vi "GetXMLTagRobust.vi"(0 "Tag only? (T)":bool=TRUE, 1 "Tag":string, 2 "String":string) -> (3 "value":string, 4 "Correct Tag Exists?":bool, 5 "tag found":string, 6 "String w/o Tag":string)   [LabVIEW 2015]
uses:
  vi.lib/regexp/Match Regular Expression.xnode
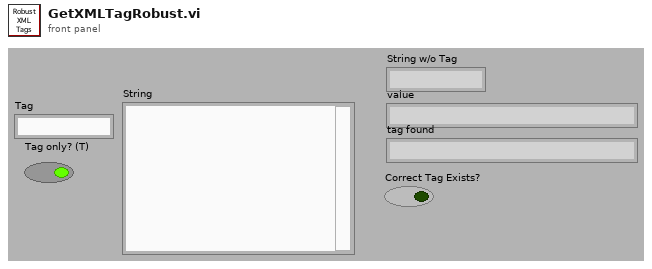
[diagram p1: front panel]
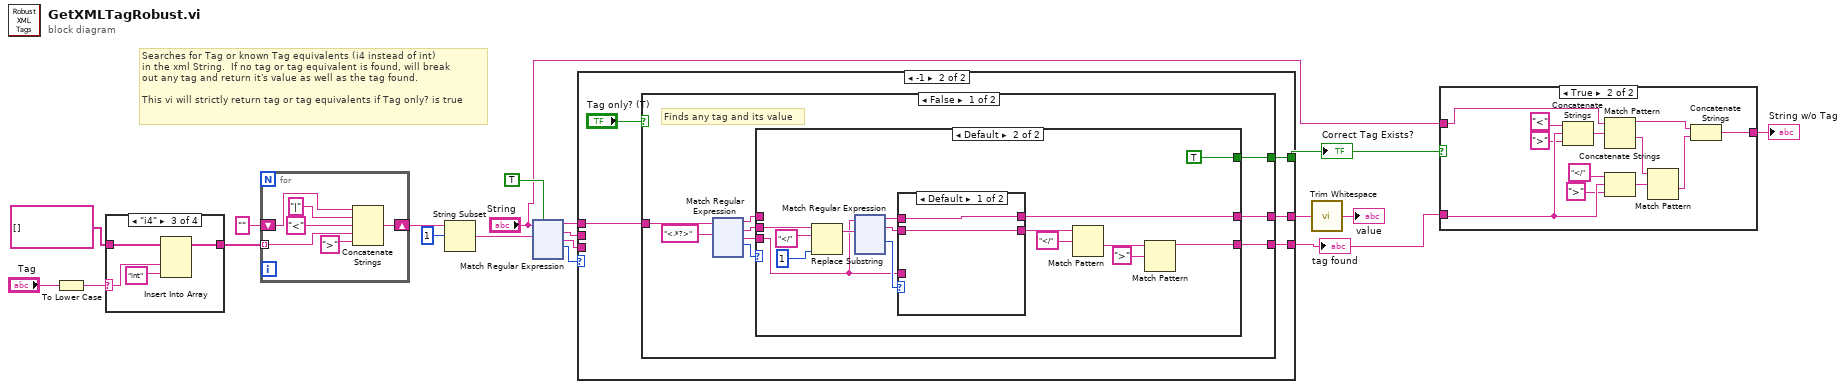
[diagram p0: block diagram]
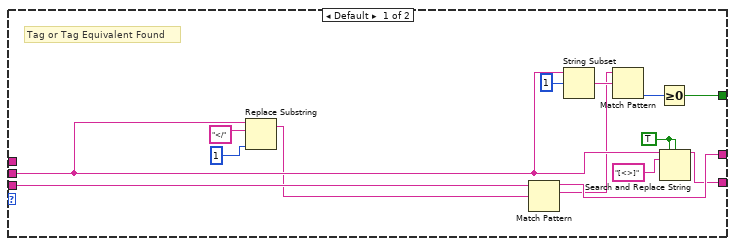
[diagram p3: hidden frame]
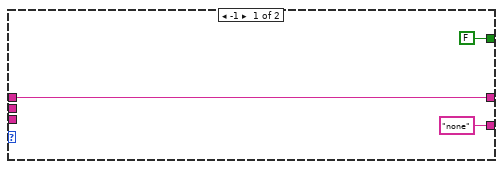
[diagram p4: hidden frame]
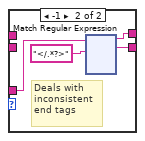
[diagram p5: hidden frame]
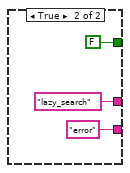
[diagram p6: hidden frame]
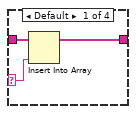
[diagram p7: hidden frame]
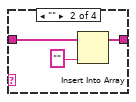
[diagram p8: hidden frame]
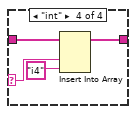
[diagram p9: hidden frame]
diagram:
  # "Searches for Tag or known Tag equivalents (i4 instead of int)\nin the xml String.  If no tag or tag equivalent is found, will break\nout any tag and return it's value as well as the tag found.\n\nThis vi will strictly return tag or tag equivalents if Tag only? is true"
  n1 = To Lower Case(string="Tag") -> (all lower case string=w7:string)
  n2 = case shown="\"i4\"" w7 {
    selector: w7 -> [w20 _ w26 w30]
    tunnel: string[] [] -> [w22 w25 w29 w33]
    tunnel: [w21 w24 w28 w32] -> w18
    frame Default {
      n3 = Insert Into Array(array=w22, new element=w20) -> (w21:string[])  [unwired: 1 in]
    }
    frame "" {
      n4 = Insert Into Array(array=w25, new element="" ("new element/subarray")) -> (w24:string[])  [unwired: 1 in]
    }
    frame "i4" {
      n5 = Insert Into Array(array=w29, new element #1=w26, new element #2="int" ("new element/subarray")) -> (w28:string[])  [unwired: 1 in]
    }
    frame "int" {
      n6 = Insert Into Array(array=w33, new element #1=w30, new element #2="i4" ("new element/subarray")) -> (w32:string[])  [unwired: 1 in]
    }
  }
  n7 = for {
    tunnel: w18 -> [w36] mode=indexing
    shift-right: [w37] -> w16
    shift-left: "" -> [w39]
    n8 = Concatenate Strings(w39, "|" ("string"), "<" ("string"), w36, ">" ("string")) -> (w37:string)
  }
  n9 = String Subset(string=w16, offset (0)=1) -> (substring=w14:string)  [unwired: 1 in]
  n10 = xnode "Match Regular Expression"("input string"="String", "regular expression"=w14, "ignore case? (F)"=TRUE) -> ("before match"=w13:string, "whole match"=w10:string, "after match"=w9:string, "offset past match"=w12:i32)  [unwired: 3 in, 1 out]
  n11 = case shown="-1" w12 {
    tunnel: w13 -> [_ w58]
    tunnel: w10 -> [w42 _]
    tunnel: w9 -> [w50 _]
    tunnel: [w53 w57] -> w6
    tunnel: [w49 w56] -> w1
    tunnel: [w51 w55] -> w4
    frame Default {
      w47 = TRUE ("replace all? (F)")
      # "Tag or Tag Equivalent Found"
      n12 = Replace Substring(2:1 ("length (len. of substring)"), 4:"</" ("substring (\"\")"), 5:w42) -> (1:w41:string)  [unwired: 1 in, 1 out]
      n13 = Match Pattern(string=w50, regular expression=w41) -> (before substring=w53:string, match substring=w40:string)  [unwired: 1 in, 2 out]
      n14 = String Subset(string=w42, offset (0)=1) -> (substring=w45:string)  [unwired: 1 in]
      n15 = Match Pattern(string=w40, regular expression=w45) -> (offset past match=w52:i32)  [unwired: 1 in, 3 out]
      n16 = Greater Or Equal To 0?(x=w52) -> (x >= 0?=w51:bool)
      n17 = Search and Replace String(replace all?=w47, case sensitive?=w47, input string=w42, search string="[<>]") -> (result string=w49:string)  [unwired: 4 in, 3 out]
    }
    frame -1 {
      n18 = case shown="False" "Tag only? (T)" {
        tunnel: w58 -> [w66 _]
        tunnel: [w63 "lazy_search" ("before match")] -> w57
        tunnel: [w62 "error" ("whole match")] -> w56
        tunnel: [w60 FALSE] -> w55
        frame False {
          # "Finds any tag and its value"
          n19 = xnode "Match Regular Expression"("input string"=w66, "regular expression"="<.*?>") -> ("before match"=w61:string, "whole match"=w59:string, "after match"=w65:string, "offset past match"=w64:i32)  [unwired: 4 in, 1 out]
          n20 = case shown="Default" w64 {
            tunnel: w65 -> [_ w75]
            tunnel: [w69 w74] -> w63
            tunnel: ["none" ("whole match") w82] -> w62
            tunnel: w61 -> [w69 _]
            tunnel: [FALSE TRUE] -> w60
            tunnel: w59 -> [_ w80]
            frame -1 {
            }
            frame Default {
              n21 = Replace Substring(2:1 ("length (len. of substring)"), 4:"</" ("substring (\"\")"), 5:w80) -> (1:w77:string)  [unwired: 1 in, 1 out]
              n22 = xnode "Match Regular Expression"("input string"=w75, "regular expression"=w77) -> ("before match"=w72:string, "whole match"=w71:string, "offset past match"=w76:i32)  [unwired: 4 in, 2 out]
              n23 = case shown="Default" w76 {
                tunnel: w75 -> [_ w91]
                tunnel: [w87 w89] -> w74
                tunnel: [w86 w88] -> w73
                tunnel: w72 -> [w87 _]
                tunnel: w71 -> [w86 _]
                frame Default {
                }
                frame -1 {
                  # "Deals with\ninconsistent \nend tags"
                  n24 = xnode "Match Regular Expression"("input string"=w91, "regular expression"="</.*?>") -> ("before match"=w89:string, "whole match"=w88:string)  [unwired: 4 in, 3 out]
                }
              }
              n25 = Match Pattern(string=w73, regular expression="</") -> (after substring=w84:string)  [unwired: 1 in, 3 out]
              n26 = Match Pattern(string=w84, regular expression=">") -> (before substring=w82:string)  [unwired: 1 in, 3 out]
            }
          }
        }
        frame True {
        }
      }
    }
  }
  "Correct Tag Exists?" <- w4
  "tag found" <- w1
  n27 = call "Trim Whitespace.vi"("string"=w6) -> ("trimmed string"=→"value":string)  [unwired: 1 in]
  n28 = case shown="True" w4 {
    tunnel: "String" -> [w428 w435]
    tunnel: w1 -> [_ w440]
    tunnel: [w428 w429] -> w2
    frame False {
    }
    frame True {
      n29 = Concatenate Strings("<" ("string"), w440, ">" ("string")) -> (w434:string)
      n30 = Match Pattern(string=w435, regular expression=w434) -> (before substring=w431:string, after substring=w433:string)  [unwired: 1 in, 2 out]
      n31 = Concatenate Strings("</" ("string"), w440, ">" ("string")) -> (w432:string)
      n32 = Match Pattern(string=w433, regular expression=w432) -> (after substring=w430:string)  [unwired: 1 in, 3 out]
      n33 = Concatenate Strings(w431, w430) -> (w429:string)
    }
  }
  "String w/o Tag" <- w2
